vi "Update Protection Signals.vi"(8 "error in (no error)":errorcluster, 9 "Overrides":dbl[](array[numeric]), 10 "Protections":T1, 11 "Frame Settings in":T2 {"Protection Configurations"."CRC Channels"."Data Type" items=["Signed", "Unsigned", "IEEE Float"]}) -> (0 "error out":errorcluster, 3 "Frame Settings out":T2 {"Protection Configurations"."CRC Channels"."Data Type" items=["Signed", "Unsigned", "IEEE Float"]})   [LabVIEW 2023, in "Protection and Counter Support Engine.lvlib"]
uses:
  Protection and Counter Support Engine.lvlib
  Types/RT Frame Settings.ctl
  Shared/Types/Exported Frame Type.ctl
  Types/RT Protection Configuration.ctl
  Shared/Types/Protection Type.ctl
  Shared/Types/XNET Signal Configuration.ctl
  Shared/Types/Exported Counter Settings.ctl
  Shared/Types/Exported Event Trigger Type.ctl
  <vilib>/NI/NIVS Inline Async API/_Data Access Engine/Data Access Engine/Types/Write.DVR.ctl
  <vilib>/NI/NIVS Inline Async API/_Data Access Engine/Access Type Classes/Write/Write.lvclass
  <vilib>/NI/NIVS Inline Async API/_Data Access Engine/Access Type Classes/Write/Write.lvclass/Write.ctl
  <vilib>/NI/NIVS Inline Async API/_Data Access Engine/Data Access Engine/Methods/Data.Processes.Execute.vi
  <vilib>/NI/NIVS Inline Async API/_Data Access Engine/Data Access Engine/Methods/Write.Data.Buffer.vi
  Get Protection Signals.vi
  <vilib>/NI/NIVS Inline Async API/_Data Access Engine/Access Type Classes/Write/Write.Buffer.vi
  <vilib>/xnet/xnet.llb/XNET Convert.vi
  <vilib>/xnet/xnet.llb/XNET Convert (Signal to Frame Raw).vi
  LP_CRC/CRC_Key_Map.vi
  LP_CRC/CRC_Calc.vi
  Shared/Protection and Counter Support Shared.lvlib
  <vilib>/NI/NIVS Inline Async API/_Data Access Engine/Data Access Engine/Data Access Engine.lvclass
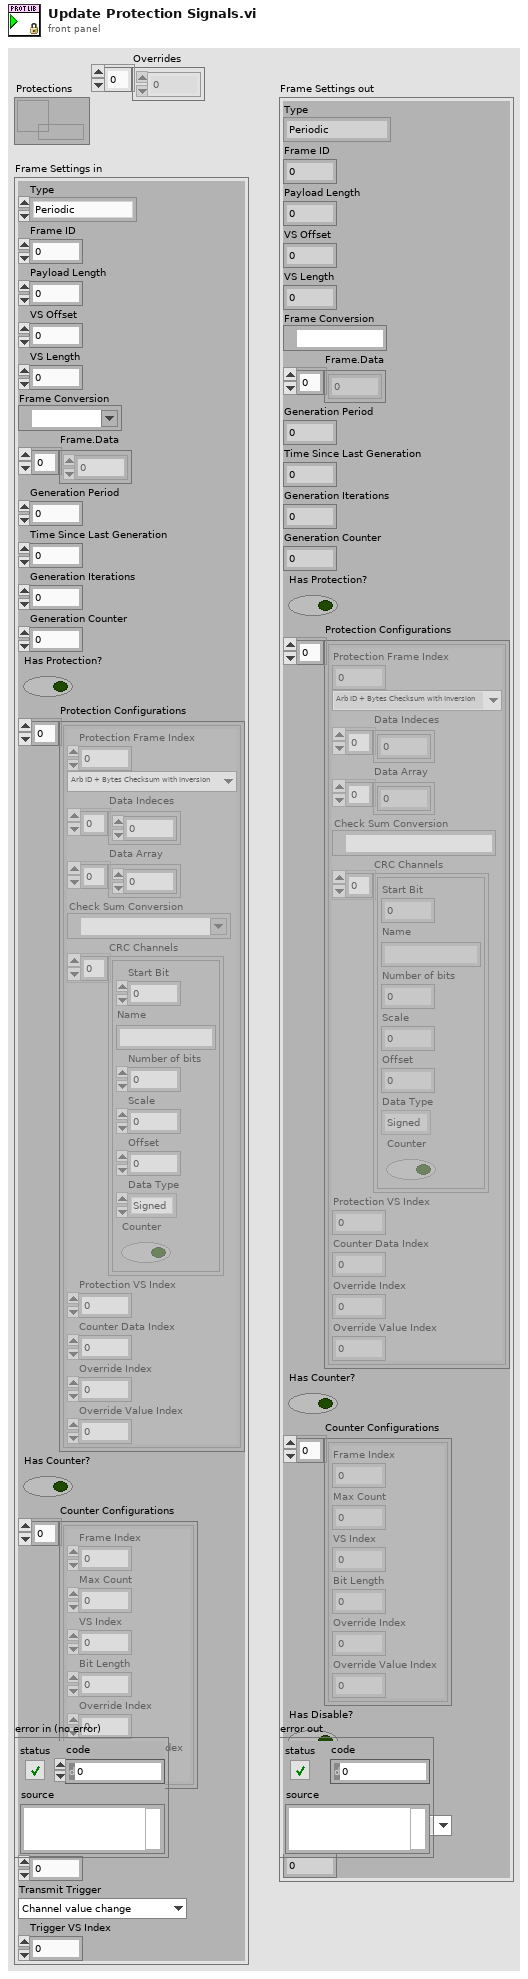
[diagram p1: front panel]
types:
  T1 = typedef "Data Access Engine.lvlib/Data Access Engine.lvclass/Write.DVR.ctl" = refnum<data-value>
  T2 = typedef "Protection and Counter Support Engine.lvlib/RT Frame Settings.ctl" = cluster{"Type":T3, "Frame ID":u32, "Payload Length":u32, "VS Offset":i32, "VS Length":i32, "Frame Conversion":refnum<k21>, "Frame.Data":dbl[], "Generation Period":u32, "Time Since Last Generation":u32, "Generation Iterations":u32, "Generation Counter":u32, "Has Protection?":bool, "Protection Configurations":T4[], "Has Counter?":bool, "Counter Configurations":T7[], "Has Disable?":bool, "Disable VS Index":i32, "Transmit Trigger":T8, "Trigger VS Index":i32}
  T3 = typedef "Protection and Counter Support Shared.lvlib/Exported Frame Type.ctl" = enum16{"Periodic", "Event", "Periodic/Event"}
  T4 = typedef "Protection and Counter Support Engine.lvlib/RT Protection Configuration.ctl" = cluster{"Protection Frame Index":i32, "Protection Type":T5, "Data Indeces":i32[], "Data Array":dbl[], "Check Sum Conversion":refnum<k21>, "CRC Channels":T6[], "Protection VS Index":i32, "Counter Data Index":i32, "Override Index":i32, "Override Value Index":i32}
  T5 = typedef "Protection and Counter Support Shared.lvlib/Protection Type.ctl" = enum16{"Arb ID + Bytes Checksum with Inversion", "Arb ID + Bytes CRC with Inversion", "Reversed Raw Signal Checksum with Inversion", "Concatenated Two's Compliment", "LP_CRC8"}
  T6 = typedef "Protection and Counter Support Shared.lvlib/XNET Signal Configuration.ctl" = cluster{"Start Bit":i32, "Name":string, "Number of bits":i32, "Scale":dbl, "Offset":dbl, "Data Type":u32, "Counter":bool}
  T7 = typedef "Protection and Counter Support Shared.lvlib/Exported Counter Settings.ctl" = cluster{"Frame Index":i32, "Max Count":dbl, "VS Index":i32, "Bit Length":i64, "Override Index":i32, "Override Value Index":i32}
  T8 = typedef "Protection and Counter Support Shared.lvlib/Exported Event Trigger Type.ctl" = enum16{"Channel value change", "Trigger channel (not zero)", "Channel value change or trigger channel (not zero)", "Trigger channel (any value change)", "Channel value change or trigger channel (any value change)"}
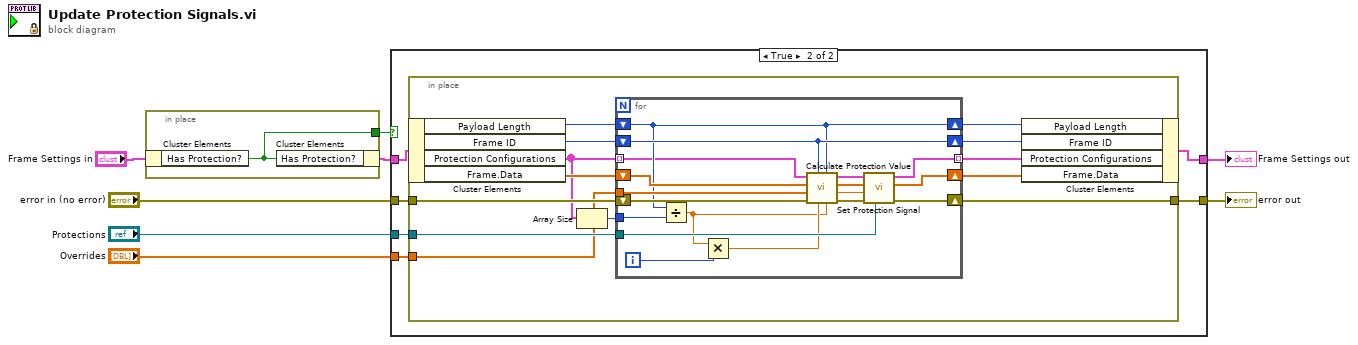
[diagram p0: block diagram]
diagram:
  n1 = in-place {
    in-place-border: [w9] -> w3
    n2 = in-place-cluster #1("Frame Settings in") -> ("Has Protection?"=w9:bool)
    n3 = in-place-cluster #1("Has Protection?"=w9) -> (w2:T2)
  }
  n4 = case shown="True" w3 {
    tunnel: "error in (no error)" -> [w11 w17]
    tunnel: [w11 w16] -> w5
    tunnel: "Protections" -> [_ w15]
    tunnel: [w10 w13] -> w8
    tunnel: w2 -> [w10 w14]
    tunnel: "Overrides" -> [_ w12]
    frame False {
    }
    frame True {
      n5 = in-place {
        in-place-border: w17 -> [w30]
        in-place-border: [w29] -> w16
        in-place-border: w15 -> [w28]
        in-place-border: w12 -> [w20]
        n6 = in-place-cluster #2(w14) -> ("Payload Length"=w25:u32, "Frame ID"=w24:u32, "Protection Configurations"=w18:T4[], "Frame.Data"=w27:dbl[])
        n7 = Array Size(array=w18) -> (size(s)=w19:i32)
        n8 = for {
          tunnel: w18 -> [w35] mode=indexing
          shift-right: [w45] -> w29
          shift-left: w30 -> [w48]
          shift-right: [w39] -> w26
          shift-left: w27 -> [w41]
          tunnel: w28 -> [w38]
          tunnel: [w42] -> w21 mode=indexing
          shift-right: [w36] -> w23
          shift-left: w25 -> [w36]
          shift-right: [w47] -> w22
          shift-left: w24 -> [w47]
          tunnel: w20 -> [w37]
          tunnel: w19 -> [w34]
          i -> [w33]
          n9 = Divide(x=w36, y=w34) -> (x/y=w31:dbl)
          n10 = Multiply(x=w31, y=w33) -> (x*y=w32:dbl)
          n11 = call "Calculate Protection Value.vi"("length"=w31, "Payload Length"=w36, "offset"=w32, "Frame ID"=w47, "error in (no error)"=w48, "Overrides"=w37, "Frame.Data in"=w41, "Protection Configuration in"=w35) -> ("error out"=w46:errorcluster, "Protection Value"=w40:dbl, "Frame.Data out"=w43:dbl[], "Protection Configuration out"=w44:T4)
          n12 = call "Set Protection Signal.vi"("Protections"=w38, "error in (no error)"=w46, "Protection Value"=w40, "Frame.Data in"=w43, "Protection Configuration in"=w44) -> ("error out"=w45:errorcluster, "Frame.Data out"=w39:dbl[], "Protection Configuration out"=w42:T4)  [unwired: 4 in]
        }
        n13 = in-place-cluster #2("Payload Length"=w23, "Frame ID"=w22, "Protection Configurations"=w21, "Frame.Data"=w26) -> (w13:T2)
      }
    }
  }
  "Frame Settings out" <- w8
  "error out" <- w5
